vi "ws Open Application Reference.vi"(8 "error in (no error)":errorcluster) -> (0 "error out":errorcluster, 3 "application reference":refnum<vi>)   [LabVIEW 2011]
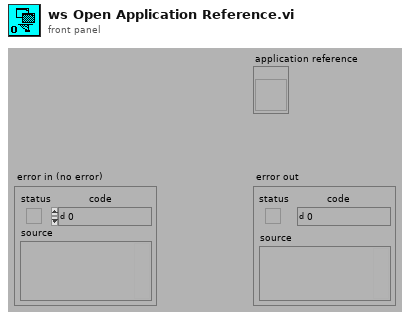
[diagram p1: front panel]
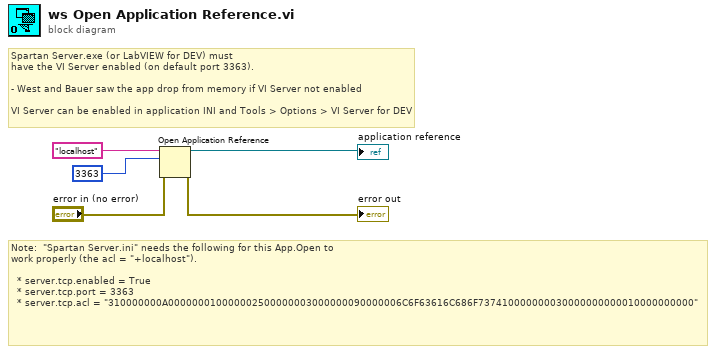
[diagram p0: block diagram]
diagram:
  # "Note:  \"Spartan Server.ini\" needs the following for this App.Open to\nwork properly (the acl = \"+localhost\").\n\n  * server.tcp.enabled = True\n  * server.tcp.port = 3363\n  * server.tcp.acl = \"310000000A000000010000002500000003000000090000006C6F63616C686F737410000000030000000000010000000000\""
  # "Spartan Server.exe (or LabVIEW for DEV) must\nhave the VI Server enabled (on default port 3363).\n\n- West and Bauer saw the app drop from memory if VI Server not enabled\n\nVI Server can be enabled in application INI and Tools > Options > VI Server for DEV"
  n1 = Open Application Reference(8:"error in (no error)", 10:u16 3363 ("port number or service name (3363)"), 11:"localhost") -> (0:→"error out":errorcluster, 3:→"application reference":refnum<vi>)  [unwired: 1 in]
